vi "log.vi"(8 "error in (no error)":errorcluster, 10 "logLineIn":string, 11 "Protocol_Generic in":refnum<class "Protocol_Generic.lvclass">) -> (0 "error out":errorcluster, 3 "Protocol_Generic out":refnum<class "Protocol_Generic.lvclass">)   [LabVIEW 2011, in "Protocol_Generic.lvclass"]
uses:
  Protocol_Generic.lvclass
  Protocol_Generic.lvclass/Protocol_Generic.ctl
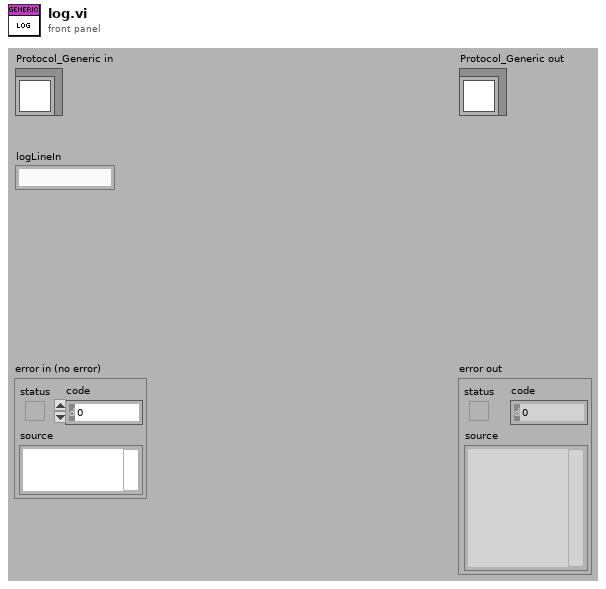
[diagram p1: front panel]
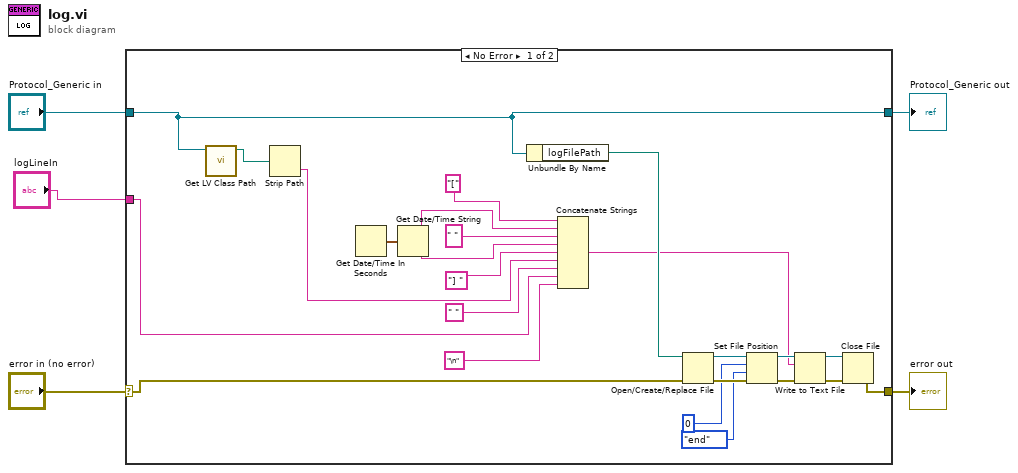
[diagram p0: block diagram]
diagram:
  n1 = case shown="No Error" "error in (no error)" {
    selector: "error in (no error)" -> [w6 w31]
    tunnel: [w22 w31] -> w4
    tunnel: [w12 w30] -> w2
    tunnel: "Protocol_Generic in" -> [w12 w30]
    tunnel: "logLineIn" -> [w9 _]
    frame No Error {
      n2 = call <vilib>:"Get LV Class Path.vi"("object"=w12) -> ("class path"=w11:path)  [unwired: 9 in, 1 out]
      n3 = Strip Path(path=w11) -> (name=w10:string)  [unwired: 1 out]
      n4 = Get Date/Time In Seconds() -> (seconds since 1Jan1904=w19:timestamp)
      n5 = Get Date/Time String(seconds (now)=w19) -> (date string=w15:string, time string=w17:string)  [unwired: 2 in]
      n6 = Unbundle By Name(w12) -> ("logFilePath"=w29:path)
      n7 = Concatenate Strings("[" ("string"), w15, " " ("string"), w17, "] " ("string"), w10, " " ("string"), w9, "\n" ("string")) -> (w18:string)
      n8 = Open/Create/Replace File(file path (use dialog)=w29, error in=w6) -> (refnum out=w26:refnum<file>, error out=w28:errorcluster)  [unwired: 4 in, 1 out]
      n9 = Set File Position(offset (in bytes) (0)=i64 0, refnum=w26, from (0:start)=enum16{"start", "end", "current"}."end", error in=w28) -> (refnum out=w25:refnum<file>, error out=w27:errorcluster)
      n10 = Write to Text File(file (use dialog)=w25, text=w18, error in=w27) -> (refnum out=w21:refnum<file>, error out=w23:errorcluster)  [unwired: 1 in, 1 out]
      n11 = Close File(refnum=w21, error in=w23) -> (error out=w22:errorcluster)  [unwired: 1 out]
    }
    frame Error {
    }
  }
  "error out" <- w4
  "Protocol_Generic out" <- w2
